vi "Get Keithley meter settings.vi"(8 "error in (no error)":errorcluster, 10 "Initial string":string, 11 "VISA Resource Name":refnum<visa-resource-name>) -> (0 "error out":errorcluster, 2 "Parameters":string, 3 "VISA Resource Name Out":refnum<visa-resource-name>, 4 "Data titles":string[](array[string])=["Signal"])   [LabVIEW 2015]
uses:
  GPIB/VISA  Send Receive.vi
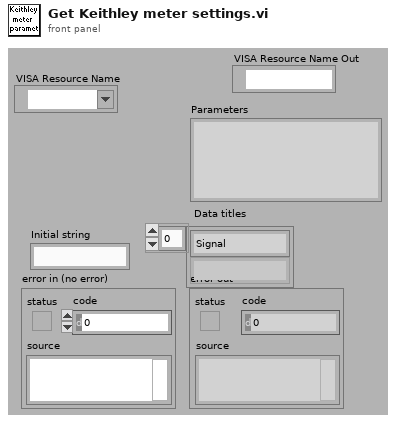
[diagram p1: front panel]
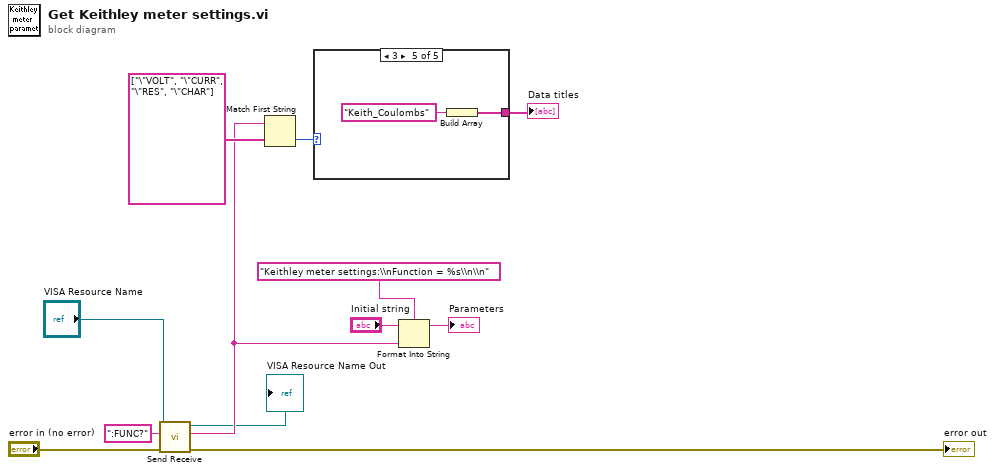
[diagram p0: block diagram]
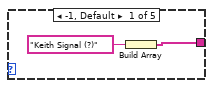
[diagram p2: hidden frame]
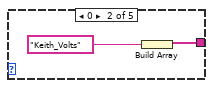
[diagram p3: hidden frame]
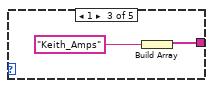
[diagram p4: hidden frame]
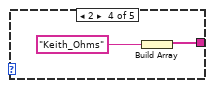
[diagram p5: hidden frame]
diagram:
  n1 = call-poly "Send Receive.vi"("error in (no error)"="error in (no error)", "data string in"=":FUNC?", "VISA Resource Name"="VISA Resource Name") -> ("error out"=→"error out":errorcluster, "data string out"=w5:string, "VISA Resource Name Out"=→"VISA Resource Name Out":refnum<visa-resource-name>)  [unwired: 6 in]
  n2 = Match First String(2:string[] ["\"VOLT", "\"CURR", "\"RES", "\"CHAR"], 3:w5) -> (0:w4:i32)  [unwired: 1 out]
  n3 = case shown="3" w4 {
    tunnel: [w14 w15 w17 w19 w21] -> w7
    frame -1, Default {
      n4 = Build Array("Keith Signal (?)") -> (w14:string[])
    }
    frame 0 {
      n5 = Build Array("Keith_Volts") -> (w15:string[])
    }
    frame 1 {
      n6 = Build Array("Keith_Amps") -> (w17:string[])
    }
    frame 2 {
      n7 = Build Array("Keith_Ohms") -> (w19:string[])
    }
    frame 3 {
      n8 = Build Array("Keith_Coulombs") -> (w21:string[])
    }
  }
  "Data titles" <- w7
  n9 = Format Into String(format string="Keithley meter settings:\\nFunction = %s\\n\\n", initial string="Initial string", w5) -> (resulting string=→"Parameters":string)  [unwired: 1 in, 1 out]
